vi "Get XNET Properties.vi"(8 "error in (no error)":errorcluster, 11 "Custom Device ref in":refnum<k24>) -> (0 "error out":errorcluster, 2 "J1939 XNET Settings":T1={"XNET Database"="", "XNET Cluster"="", "CAN Port"="", "Baud rate [Bd]"=0, "Termination"=0, "Incoming Rate"=0, "Outcoming Rate"=0, "Write Decimation"=100} {"Termination" items=["Off", "On"]}, 3 "Custom Device ref out":refnum<k24>)   [LabVIEW 2013, in "J1939 System Definition API Support.lvlib"]
uses:
  J1939 System Definition API Support.lvlib
  NationalInstruments.VeriStand.SystemDefinitionAPI
  Shared/Types/XNET Settings.ctl
  Shared/SubVIs/Constants.vi
  <vilib>/NI Veristand/Custom Device API/Get Item Property (Variant).vi
  Shared/J1939 Addon Shared.lvlib
  <vilib>/NI Veristand/Custom Device API/Custom Device API.lvlib
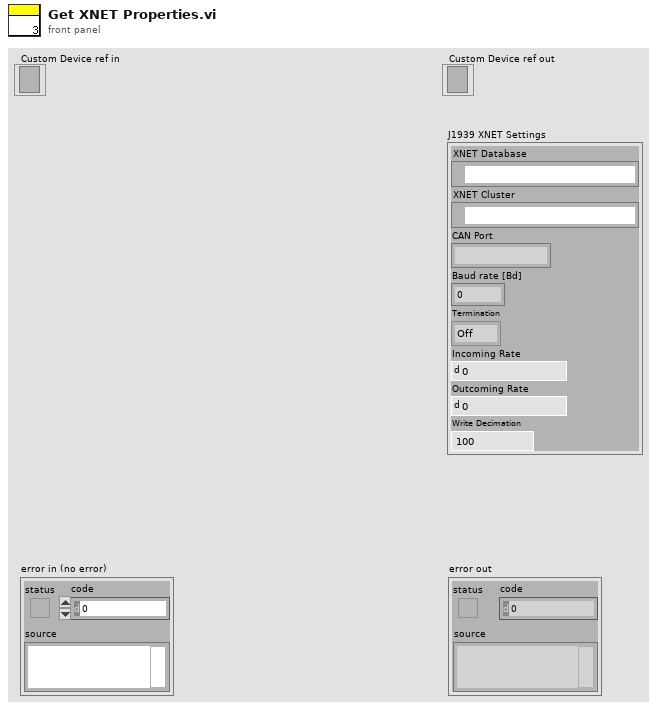
[diagram p1: front panel]
types:
  T1 = typedef "J1939 Addon Shared.lvlib/XNET Settings.ctl" = cluster{"XNET Database":refnum<k21>, "XNET Cluster":refnum<k21>, "CAN Port":string, "Baud rate [Bd]":u32, "Termination":u32, "Incoming Rate":u32, "Outcoming Rate":u32, "Write Decimation":u32}
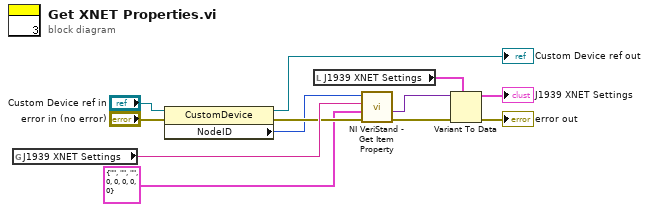
[diagram p0: block diagram]
diagram:
  n1 = global read "Constants.vi" "J1939 XNET Settings"() -> (w9:string)
  n2 = property class="CustomDevice"(reference="Custom Device ref in", error in="error in (no error)") -> (reference out=→"Custom Device ref out":refnum<k24>, error out=w8:errorcluster, "NodeID"=w7:u64)
  n3 = local read "J1939 XNET Settings"() -> (w3:T1)
  n4 = call-poly <vilib>:"NI VeriStand - Get Item Property.vi"("error in (no error)"=w8, "Default Value"=T1 {"XNET Database"="", "XNET Cluster"="", "CAN Port"="", "Baud rate [Bd]"=0, "Termination"=0, "Incoming Rate"=0, "Outcoming Rate"=0, "Write Decimation"=0} ("J1939 XNET Settings"), "Property Name"=w9, "Item Ref in"=w7) -> ("error out"=w6:errorcluster, "Value"=w4:variant)  [unwired: 4 in, 2 out]
  n5 = Variant To Data(error in=w6, type=w3, Variant=w4) -> (data=→"J1939 XNET Settings":T1, error out=→"error out":errorcluster)
